vi "CustomGaugeInit.vi"(3 "Container State":T3, 4 "Previous State":variant, 5 "Previous Version":T2) -> (2 "Current State":T1)   [LabVIEW 2012, in "CustomGauge.xctl"]
uses:
  CustomGauge.xctl
  CustomGaugeState.ctl
  <vilib>/_xctls/Container State.ctl
  <vilib>/_xctls/Version.ctl
  <vilib>/_xctls/XControlSupport.lvlib
panel:
  in  "Default Indicator State":T1
  in  "Default Control State":T1
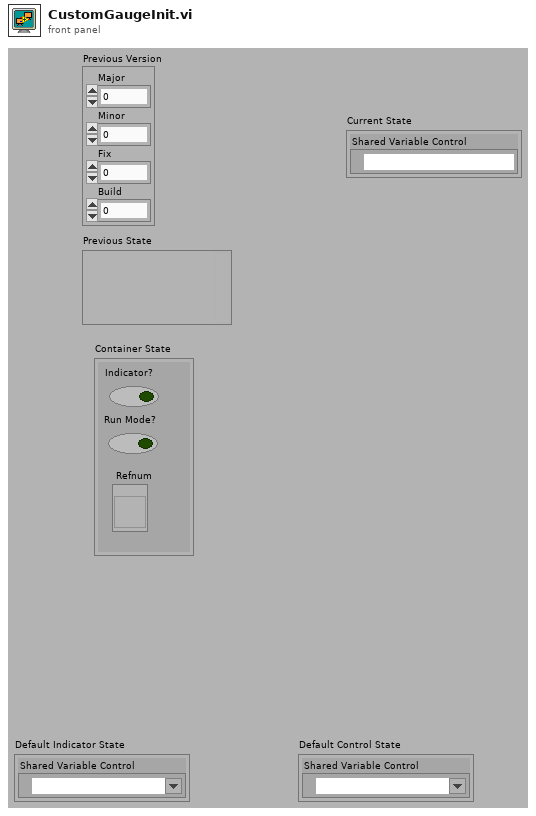
[diagram p1: front panel]
types:
  T1 = typedef "CustomGauge.xctl/CustomGaugeState.ctl" = cluster{"Shared Variable Control":refnum<k21>}
  T2 = typedef "XControlSupport.lvlib/Version.ctl" = cluster{"Major":u16, "Minor":u16, "Fix":u16, "Build":u16}
  T3 = typedef "XControlSupport.lvlib/Container State.ctl" = cluster{"Indicator?":bool, "Run Mode?":bool, " Refnum":refnum<vi>}
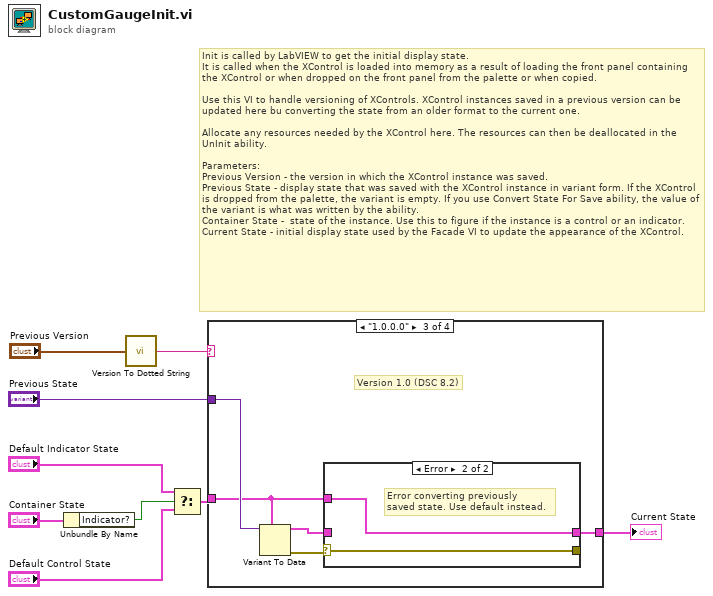
[diagram p0: block diagram]
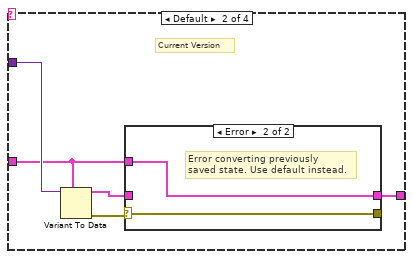
[diagram p3: hidden frame]
diagram:
  # "Init is called by LabVIEW to get the initial display state.\nIt is called when the XControl is loaded into memory as a result of loading the front panel containing the XControl or when dropped on the front panel from the palette or when copied.\n\nUse this VI to handle versioning of XControls. XControl instances saved in a previous version can be updated here bu converting the state from an older format to the current one.\n\nAllocate any resources needed by the XControl here. The resources can then be deallocated in the UnInit ability.\n\nParameters:\nPrevious Version - the version in which the XControl instance was saved.\nPrevious State - display state that was saved with the XControl instance in variant form. If the XControl is dropped from the palette, the variant is empty. If you use Convert State For Save ability, the value of the variant is what was written by the ability. \nContainer State -  state of the instance. Use this to figure if the instance is a control or an indicator.\nCurrent State - initial display state used by the Facade VI to update the appearance of the XControl."
  n1 = Unbundle By Name("Container State") -> ("Indicator?"=w4:bool)
  n2 = call <vilib>:"Version To Dotted String.vi"("Version"="Previous Version") -> ("String Version"=w1:string)
  n3 = Select(t="Default Indicator State", s=w4, f="Default Control State") -> (s? t:f=w3:T1)
  n4 = case shown="\"1.0.0.0\"" w1 {
    tunnel: "Previous State" -> [_ w15 w24 _]
    tunnel: [w10 w11 w20 w29] -> w8
    tunnel: w3 -> [w10 w12 w21 w29]
    frame "False" {
      # "Convert from previous version"
    }
    frame Default {
      # "Current Version"
      n5 = Variant To Data(type=w12, Variant=w15) -> (data=w13:T1, error out=w14:errorcluster)  [unwired: 1 in]
      n6 = case shown="Error" w14 {
        selector: w14 -> [w17 w18]
        tunnel: w13 -> [w16 _]
        tunnel: [w16 w19] -> w11
        tunnel: w12 -> [_ w19]
        tunnel: [w17 w18] -> _
        frame No Error {
        }
        frame Error {
          # "Error converting previously \nsaved state. Use default instead."
        }
      }
    }
    frame "1.0.0.0" {
      # "Version 1.0 (DSC 8.2)"
      n7 = Variant To Data(type=w21, Variant=w24) -> (data=w22:T1, error out=w23:errorcluster)  [unwired: 1 in]
      n8 = case shown="Error" w23 {
        selector: w23 -> [w26 w27]
        tunnel: w22 -> [w25 _]
        tunnel: [w25 w28] -> w20
        tunnel: w21 -> [_ w28]
        tunnel: [w26 w27] -> _
        frame No Error {
        }
        frame Error {
          # "Error converting previously \nsaved state. Use default instead."
        }
      }
    }
    frame "0.0.0.0" {
      # "Just created, use default state"
    }
  }
  "Current State" <- w8
